vi "fast_match.vi"(8 "error in (no error)":errorcluster, 10 "Template":T1, 11 "Image":T1) -> (0 "error out":errorcluster, 1 "score":dbl, 2 "y shift":i32, 3 "x shift":i32)   [LabVIEW 2016]
doc: "Passes image and template to DLL to calculate normalised cross correlation peak position and value."
uses:
  <vilib>/vision/Image Controls.llb/IMAQ Image.ctl
  template_match.dll
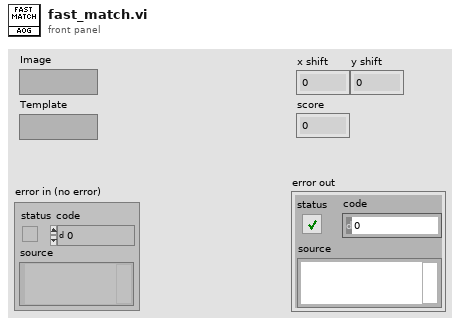
[diagram p1: front panel]
types:
  T1 = typedef "IMAQ Image.ctl" = refnum<image>
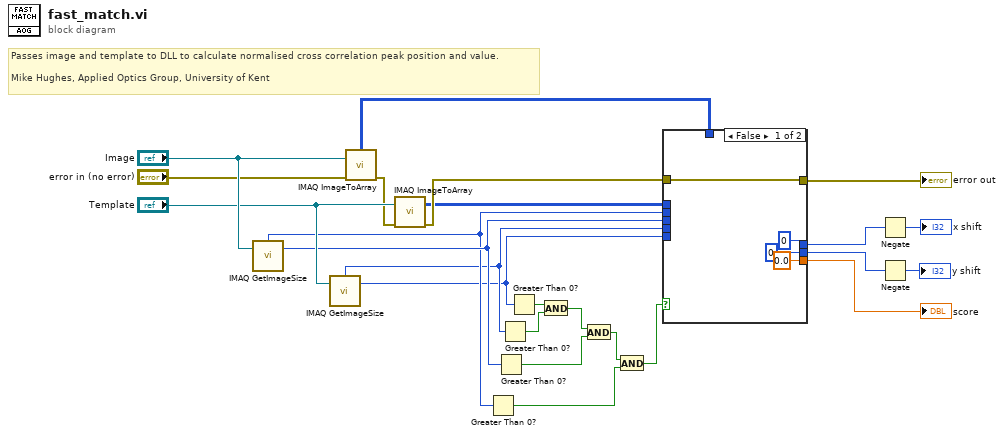
[diagram p0: block diagram]
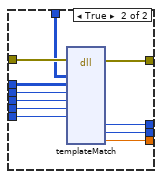
[diagram p2: hidden frame]
diagram:
  # "Passes image and template to DLL to calculate normalised cross correlation peak position and value.\n\nMike Hughes, Applied Optics Group, University of Kent"
  n1 = call "IMAQ GetImageSize"("Image"="Image") -> ("Y Resolution"=w11:i32, "X Resolution"=w10:i32)  [unwired: 3 in, 1 out]
  n2 = call "IMAQ GetImageSize"("Image"="Template") -> ("Y Resolution"=w8:i32, "X Resolution"=w9:i32)  [unwired: 3 in, 1 out]
  n3 = call "IMAQ ImageToArray"("error in (no error)"="error in (no error)", "Image"="Image") -> ("error out"=w20:errorcluster, "Image Pixels (U8)"=w13:u8[][])  [unwired: 2 in, 3 out]
  n4 = call "IMAQ ImageToArray"("error in (no error)"=w20, "Image"="Template") -> ("error out"=w19:errorcluster, "Image Pixels (U8)"=w12:u8[][])  [unwired: 2 in, 3 out]
  n5 = Greater Than 0?(x=w10) -> (x > 0?=w3:bool)
  n6 = Greater Than 0?(x=w11) -> (x > 0?=w5:bool)
  n7 = Greater Than 0?(x=w9) -> (x > 0?=w6:bool)
  n8 = Greater Than 0?(x=w8) -> (x > 0?=w7:bool)
  n9 = And(x=w7, y=w6) -> (x .and. y?=w4:bool)
  n10 = And(x=w4, y=w5) -> (x .and. y?=w2:bool)
  n11 = And(x=w2, y=w3) -> (x .and. y?=w1:bool)
  n12 = case shown="False" w1 {
    tunnel: [0.0 ("score") w39] -> w22
    tunnel: w19 -> [w28 w38]
    tunnel: [w28 w37] -> w18
    tunnel: [0 ("x_shift") w36] -> w17
    tunnel: [0 ("y_shift") w35] -> w15
    tunnel: w13 -> [_ w34]
    tunnel: w12 -> [_ w33]
    tunnel: w11 -> [_ w32]
    tunnel: w10 -> [_ w31]
    tunnel: w9 -> [_ w30]
    tunnel: w8 -> [_ w29]
    frame False {
    }
    frame True {
      n13 = dll-call lib="\\\\healey\\aog/general storage/REBOT/code/volume_assembly/Labview Raptor/Raptor3/lib/template_match.dll" fn="templateMatch"(error in=w38, "src"=w34, "templ"=w33, "src_cols"=w31, "src_rows"=w32, "templ_cols"=w30, "templ_rows"=w29) -> (error out=w37:errorcluster, "x_shift"=w36:i32, "y_shift"=w35:i32, "score"=w39:dbl)  [unwired: 12 in, 1 out]
    }
  }
  "score" <- w22
  "error out" <- w18
  n14 = Negate(x=w17) -> (-x=→"x shift":i32)
  n15 = Negate(x=w15) -> (-x=→"y shift":i32)
